vi "Configure Frequency Offset.vi"(8 "error in (no error)":errorcluster {"code" format="%.0x"}, 9 "frequency offset":dbl caption="frequency offset (Hz)", 11 "instrument handle":refnum<k15>) -> (0 "error out":errorcluster {"code" format="%.0x"}, 3 "instrument handle out":refnum<k15>)   [LabVIEW 2009, in "Keysight XSAn.lvlib"]
doc: "This VI configures the Frequency Offset property of the spectrum analyzer. This function affects the setting of the spectrum analyzer's absolute frequencies, such as start, stop, center, and marker. It does not affect values such as span and delta marker, which are the difference of frequencies.\n\nSupported Models: M9290A, N8973B, N8974B, N8975B, N8976B, N9000A, N9000B, N9010A, N9010B, N9020A, N9020B, N9030A, N9030B, N9038A, N9040B, N9041B, SPN9003A, SPN9026A"
uses:
  <instrlib>/Keysight XSAn/Keysight XSAn.lvlib
  AgXSAn.dll
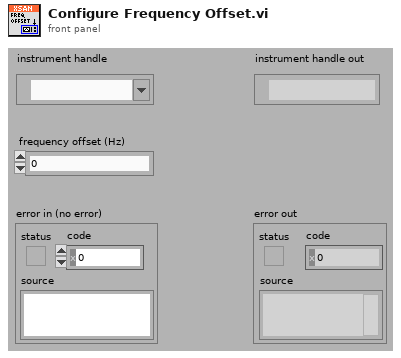
[diagram p1: front panel]
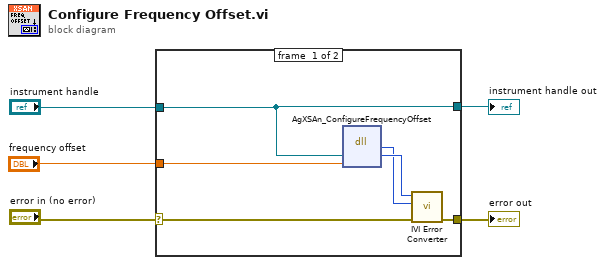
[diagram p0: block diagram]
diagram:
  n1 = case shown="No Error" "error in (no error)" {
    selector: "error in (no error)" -> [w9 w13]
    tunnel: [w10 w13] -> w4
    tunnel: "instrument handle" -> [w7 w12]
    tunnel: [w7 w12] -> w2
    tunnel: "frequency offset" -> [w6 _]
    frame #0 {
      n2 = dll-call lib="AgXSAn**.dll" fn="AgXSAn_ConfigureFrequencyOffset" ("LabVIEW:IviSpecAn_ConfigureFrequencyOffset")("instrument handle"=w7, "frequency offset"=w6) -> ("Status"=w8:i32, "instrument handle"=w11:u32)  [unwired: 4 in, 2 out]
      n3 = call <instrlib>:"IVI Error Converter.vi"("error in (no error)"=w9, "IVI error code (0)"=w8, "instrument handle"=w11) -> ("error out"=w10:errorcluster)  [unwired: 7 in, 1 out]
    }
    frame #1 {
    }
  }
  "error out" <- w4
  "instrument handle out" <- w2
